vi "LabVLC - Example.vi"(0 "Video Speed":sgl(slide)=1.002012 min=0 max=2 step=0.1 scale=0.0..2.0, 1 "Stop":bool) -> ()   [LabVIEW 2014]
doc: "The MIT License (MIT)\n\nCopyright (c) 2015 Ian McIntyre\n\nPermission is hereby granted, free of charge, to any person obtaining a copy\nof this software and associated documentation files (the \"Software\"), to deal\nin the Software without restriction, including without limitation the rights\nto use, copy, modify, merge, publish, distribute, sublicense, and/or sell\ncopies of the Software, and to permit persons to whom the Software is\nfurnished to do so, subject to the following conditions:\n\nThe above copyright notice and this permission notice shall be included in\nall copies or substantial portions of the Software.\n\nTHE SOFTWARE IS PROVIDED \"AS IS\", WITHOUT WARRANTY OF ANY KIND, EXPRESS OR\nIMPLIED, INCLUDING BUT NOT LIMITED TO THE WARRANTIES OF MERCHANTABILITY,\nFITNESS FOR A PARTICULAR PURPOSE AND NONINFRINGEMENT. IN NO EVENT SHALL THE\nAUTHORS OR COPYRIGHT HOLDERS BE LIABLE FOR ANY CLAIM, DAMAGES OR OTHER\nLIABILITY, WHETHER IN AN ACTION OF CONTRACT, TORT OR OTHERWISE, ARISING FROM,\nOUT OF OR IN CONNECTION WITH THE SOFTWARE OR THE USE OR OTHER DEALINGS IN\nTHE SOFTWARE."
uses:
  System.Windows.Forms
panel:
  in  "PictureBox":refnum<k24>(container)
  in  "Volume":i32(slide) min=0 max=100 step=1 scale=0.0..100.0
  in  "mute":bool
  in  "pause":bool
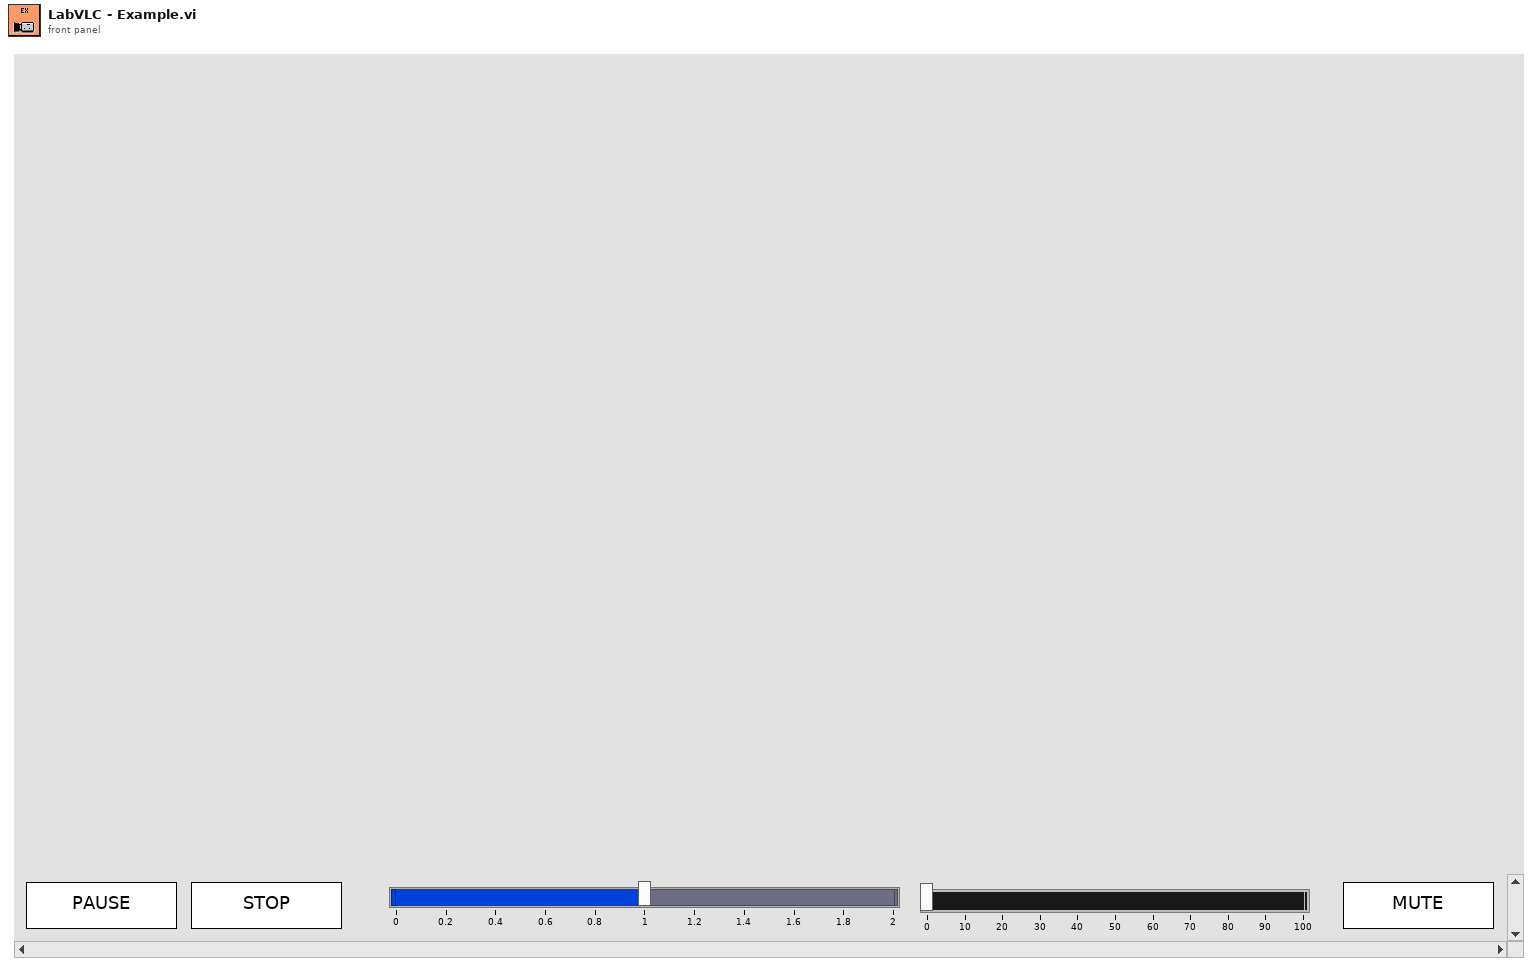
[diagram p1: front panel]
types:
  T1 = cluster{"media_ptr":i32, "vlc_inst_ptr":i32, "path in":path}
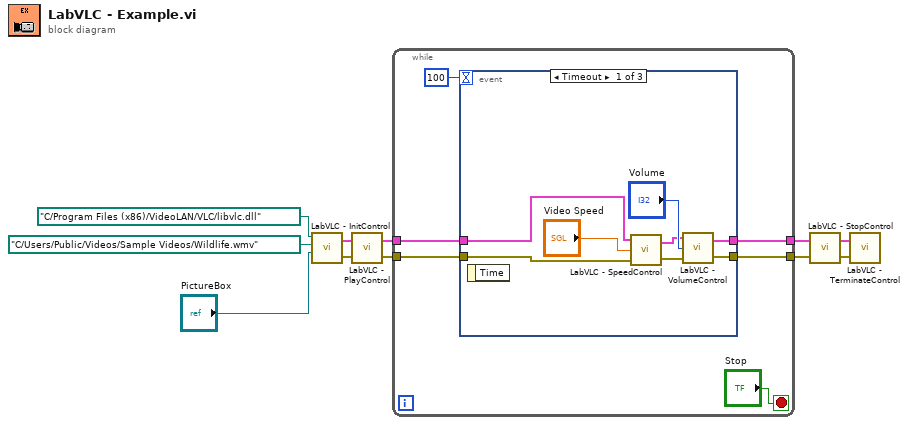
[diagram p0: block diagram]
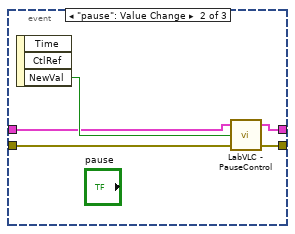
[diagram p2: hidden frame]
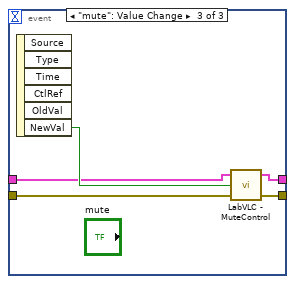
[diagram p3: hidden frame]
diagram:
  n1 = call "LabVLC - InitControl.vi"(".NET Refnum in"="PictureBox", "playback_video"=path "C:/Users/Public/Videos/Sample Videos/Wildlife.wmv", "vlc_dll_in"=path "C:/Program Files (x86)/VideoLAN/VLC/libvlc.dll" ("path in")) -> ("error out"=w9:errorcluster, "out"=w5:T1)  [unwired: 1 in]
  n2 = call "LabVLC - PlayControl.vi"("error in (no error)"=w9, "struct"=w5) -> ("error out"=w10:errorcluster, "output cluster"=w4:T1)
  n3 = while {
    tunnel: w10 -> [w16]
    tunnel: [w14] -> w8
    tunnel: [w13] -> w2
    tunnel: w4 -> [w12]
    stop <- "Stop" stop-if-true
    n4 = event shown="[0] Timeout" {
      selector: _ -> [_ _ _]
      dyn-events: _ -> [_ _ _]
      timeout: 100 -> [_ _ _]
      tunnel: w16 -> [w25 w30 w33]
      tunnel: [w22 w29 w32] -> w14
      tunnel: [w18 w28 w35] -> w13
      tunnel: w12 -> [w19 w26 w31]
      event Timeout {
        n5 = event-data() -> ()  [unwired: 1 in, 1 out]
        n6 = call "LabVLC - SpeedControl.vi"("error in (no error)"=w25, "video_speed"="Video Speed", "struct"=w19) -> ("error out"=w23:errorcluster, "out"=w20:T1)
        n7 = call "LabVLC - VolumeControl.vi"("error in (no error)"=w23, "volume (percents)"="Volume", "struct"=w20) -> ("error out"=w22:errorcluster, "out"=w18:T1)
      }
      event "pause": Value Change {
        n8 = event-data() -> ("NewVal"=w27:bool)  [unwired: 1 in, 2 out]
        n9 = call "LabVLC - PauseControl.vi"("error in (no error)"=w30, "is_paused"=w27, "struct"=w26) -> ("error out"=w29:errorcluster, "out"=w28:T1)  [unwired: 1 out]
      }
      event "mute": Value Change {
        n10 = event-data() -> ("NewVal"=w34:bool)  [unwired: 1 in, 5 out]
        n11 = call "LabVLC - MuteControl.vi"("error in (no error)"=w33, "is_mute"=w34, "struct"=w31) -> ("error out"=w32:errorcluster, "out"=w35:T1)  [unwired: 1 out]
      }
    }
  }
  n12 = call "LabVLC - StopControl.vi"("error in (no error)"=w8, "struct"=w2) -> ("error out"=w6:errorcluster, "out"=w1:T1)
  n13 = call "LabVLC - TerminateControl.vi"("error in (no error)"=w6, "struct"=w1) -> ()  [unwired: 1 in, 1 out]
